vi "Process.vi"(8 "error in":errorcluster, 11 "MAUI":refnum<class "SMO.UI.MAUI.lvclass">) -> (0 "error out":errorcluster, 3 "MAUI out":refnum<class "SMO.UI.MAUI.lvclass">)   [LabVIEW 2020, in "SMO.UI.MAUI.lvclass"]
doc: "---------------------------------------------------------------\nJKI State Machine Objects™\nhttp://jki.net/state-machine-objects/\nCopyright (C) 2005-2015, JKI <info@jki.net>\nALL RIGHTS RESERVEDJKI State Machine Objects (SMO) 1.0.0.5\nJKI - JKI\nCopyright (c) 2016, JKI"
uses:
  SMO.UI.MAUI.lvclass
  C:/Program Files (x86)/National Instruments/LabVIEW 2020/vi.lib/JKI/JKI SMO/SMO/SMO.lvclass
  C:/Program Files (x86)/National Instruments/LabVIEW 2020/vi.lib/JKI/JKI SMO/SMO.UI/SMO.UI.lvclass
  <vilib>/JKI/JKI SMO/SMO/Typedefs/Parent Call--Enum.ctl
  Typedefs/DefaultSubpanel.ctl
  <vilib>/Levylab/SMO.UI.Embedded/SMO.UI.Embedded.lvclass
  SMO.UI.MAUI.lvclass/SMO.UI.MAUI.ctl
  <vilib>/Levylab/SMO.UI.Embedded/Typedefs/UI State.ctl
  Typedefs/PublicEvents--SMO.UI.MAUI.ReadyForInfo .ctl
  <vilib>/JKI/JKI SMO/SMO.UI/SMO.UI.lvclass
  <vilib>/JKI/JKI SMO/SMO/SMO.lvclass
panel:
  out "License":string="BSD 3-Clause License\n\nCopyright (c) 2020, Joseph Albro\nAll rights reserved.\n\nRedistribution and use in source and binary forms, with or without\nmodification, are permitted provided that the following conditions are met:\n\n1. Redistributions of source code must retain the above copyright notice, this\n   list of conditions and the following disclaimer.\n\n2. Redistributions in binary form must reproduce the above copyright notice,\n   this list of conditions and the following disclaimer in the documentation\n   and/or other materials provided with the distribution.\n\n3. Neither the name of the copyright holder nor the names of its\n   contributors may be used to endorse or promote products derived from\n   this software without specific prior written permission.\n\nTHIS SOFTWARE IS PROVIDED BY THE COPYRIGHT HOLDERS AND CONTRIBUTORS \"AS IS\"\nAND ANY EXPRESS OR IMPLIED WARRANTIES, INCLUDING, BUT NOT LIMITED TO, THE\nIMPLIED WARRANTIES OF MERCHANTABILITY AND FITNESS FOR A PARTICULAR PURPOSE ARE\nDISCLAIMED. IN NO EVENT SHALL THE COPYRIGHT HOLDER OR CONTRIBUTORS BE LIABLE\nFOR ANY DIRECT, INDIRECT, INCIDENTAL, SPECIAL, EXEMPLARY, OR CONSEQUENTIAL\nDAMAGES (INCLUDING, BUT NOT LIMITED TO, PROCUREMENT OF SUBSTITUTE GOODS OR\nSERVICES; LOSS OF USE, DATA, OR PROFITS; OR BUSINESS INTERRUPTION) HOWEVER\nCAUSED AND ON ANY THEORY OF LIABILITY, WHETHER IN CONTRACT, STRICT LIABILITY,\nOR TORT (INCLUDING NEGLIGENCE OR OTHERWISE) ARISING IN ANY WAY OUT OF THE USE\nOF THIS SOFTWARE, EVEN IF ADVISED OF THE POSSIBILITY OF SUCH DAMAGE."
  # "For instructions on how to use the JKI State Machine Objects, examples and video tutorials, visit:\nhttp://jki.net/state-machine-objects/\n\nJKI State Machine Objects™\nhttp://jki.net/state-machine-objects/\nCopyright (C) 2005-2015, JKI <info@jki.net>\nALL RIGHTS RESERVED"
  # "SMO.UI.MAUI"
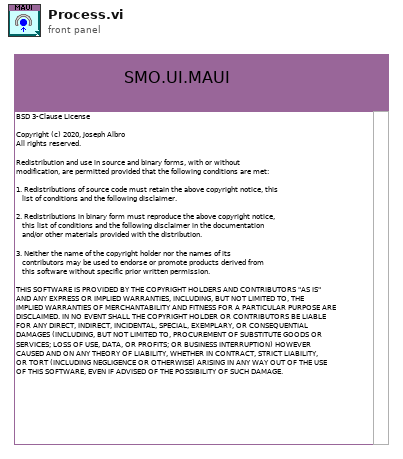
[diagram p1: front panel]
types:
  T1 = typedef "SMO.lvclass/Parent Call--Enum.ctl" = enum16{"Allows parent to run", "Does not request parent to run"}
  T2 = typedef "SMO.UI.MAUI.lvclass/DefaultSubpanel.ctl" = cluster{"SMO.UI.Embedded":refnum<class "SMO.UI.Embedded.lvclass">}
  T3 = enum32{"invalid app kind", "Development System", "Run Time System", "Student Edition", "Embedded LabVIEW", "Evaluation", "Custom"}
  T4 = enum32{"Invalid", "Standard", "Closed", "Hidden", "Minimized", "Maximized"}
  T5 = typedef "SMO.UI.MAUI.lvclass/PublicEvents--SMO.UI.MAUI.ReadyForInfo .ctl" = bool
  T6 = typedef "SMO.UI.MAUI.lvclass/PrivateEvents--SMO.UI.MAUI.GetDefaultSubpanel.ctl" = refnum<notifier>
  T7 = cluster{"SMO.UI.Embedded":refnum<class "SMO.UI.Embedded.lvclass">}
  T8 = typedef "SMO.UI.Embedded.lvclass/UI State.ctl" = enum16{"unknown", "Opened", "Embedded", "Closed"}
  T9 = cluster{"Core":cluster{"Current VI Reference":refnum<vi>, "Close Panel on Exit?":bool, "error":errorcluster}, "Self Reference":refnum<class "SMO.UI.MAUI.lvclass">, "Active Index":i32[], "Panel Index":i32[], "UI State":T8, "PopSubpanel":i32}
  T10 = typedef "SMO.UI.MAUI.lvclass/PrivateEvents--SMO.UI.MAUI.OpenSubpanel.ctl" = i32
  T11 = typedef "SMO.UI.MAUI.lvclass/PrivateEvents--SMO.UI.MAUI.SetPanelData.ctl" = T12[]
  T12 = typedef "SMO.UI.MAUI.lvclass/PanelData.ctl" = cluster{"SubPanel":refnum<vi>, "Ring":refnum<vi>, "Active":i32}
  T13 = typedef "SMO.UI.MAUI.lvclass/PrivateEvents--SMO.UI.MAUI.GetPanelData.ctl" = refnum<notifier>
  T14 = cluster{"Current VI Reference":refnum<vi>, "Close Panel on Exit?":bool, "error":errorcluster}
  T15 = typedef "SMO.lvclass/Protected Events.ctl" = cluster{"StopProcesses":refnum<user-event>, "AbortProcesses":refnum<user-event>, "Config Changed":refnum<user-event>, "Dependency":refnum<user-event>}
  T16 = typedef "SMO.UI.MAUI.lvclass/PrivateEvents--Cluster.ctl" = cluster{"SetEmbedded":refnum<user-event>, "GetEmbedded":refnum<user-event>, "SetPanelData":refnum<user-event>, "GetPanelData":refnum<user-event>, "UpdatePanel":refnum<user-event>, "PopSubpanel":refnum<user-event>, "GetDefaultSubpanel":refnum<user-event>, "SetDefaultSubpanel":refnum<user-event>}
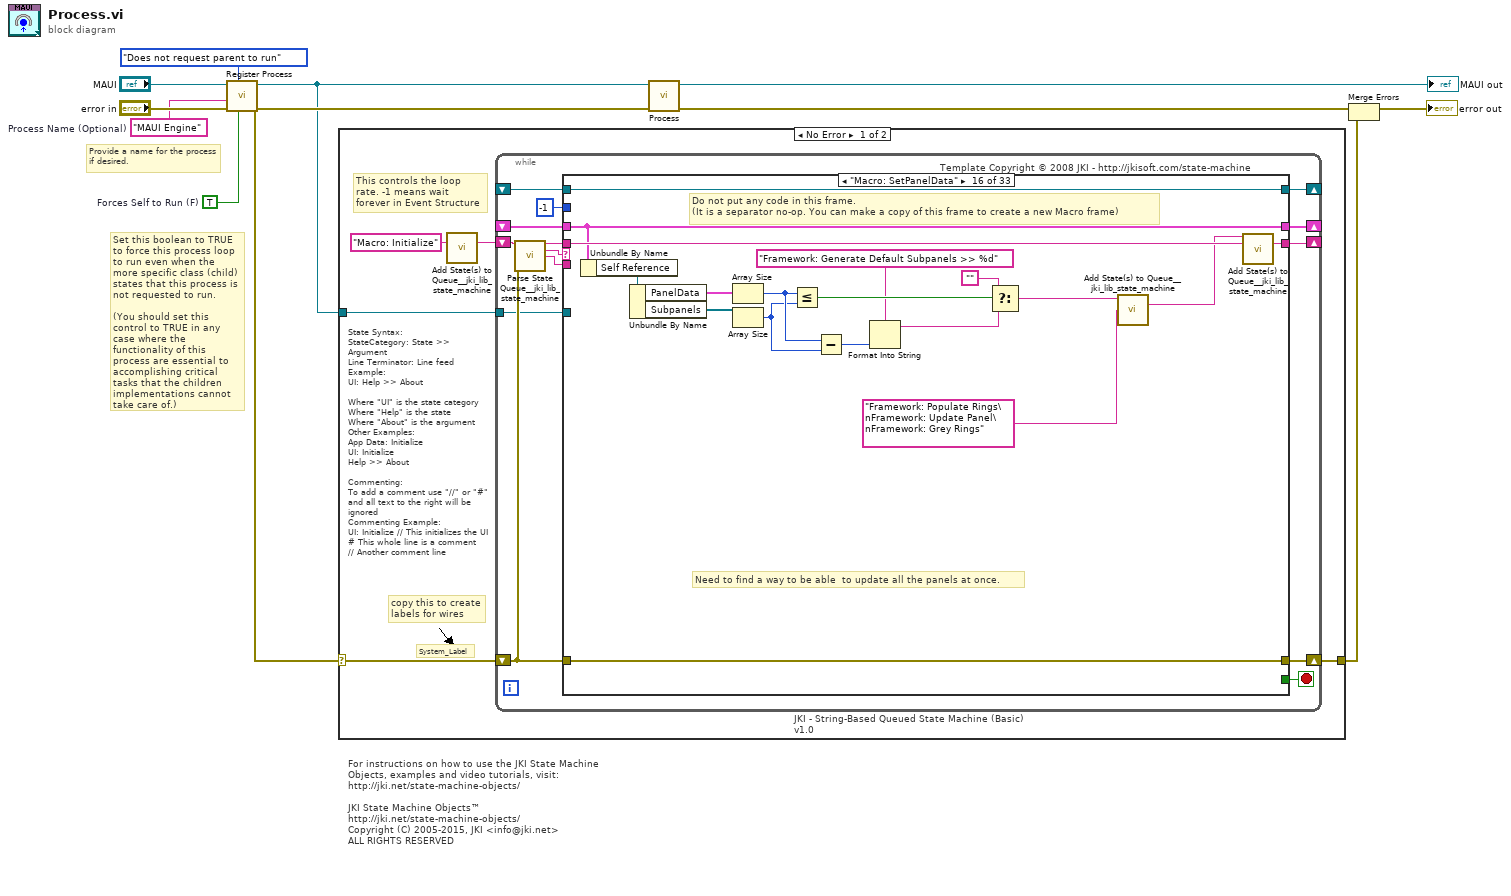
[diagram p0: block diagram]
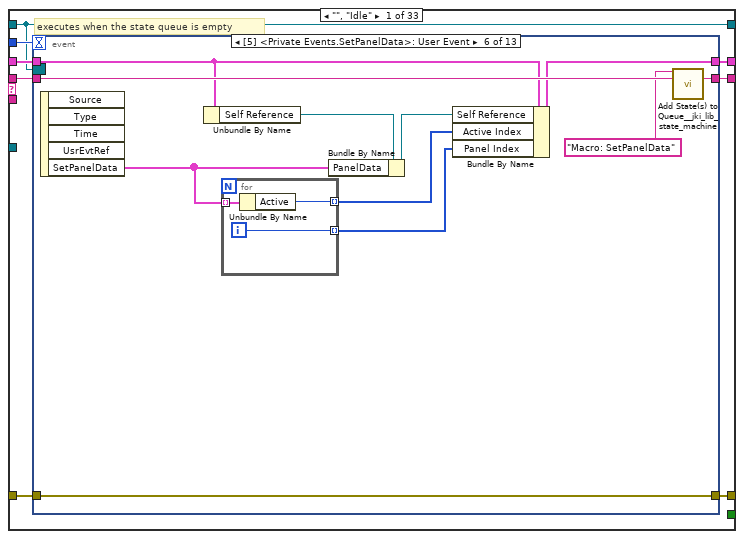
[diagram p2: hidden frame]
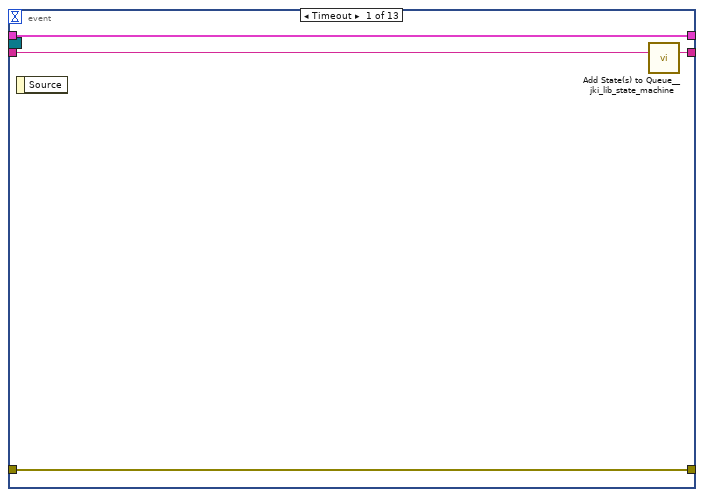
[diagram p3: hidden frame]
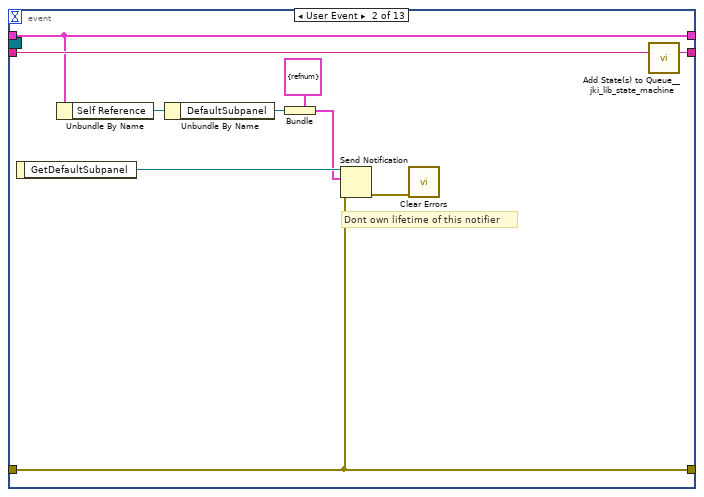
[diagram p4: hidden frame]
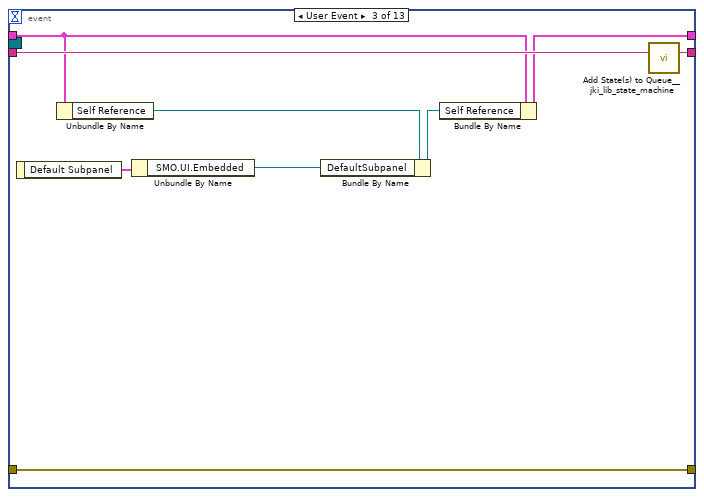
[diagram p5: hidden frame]
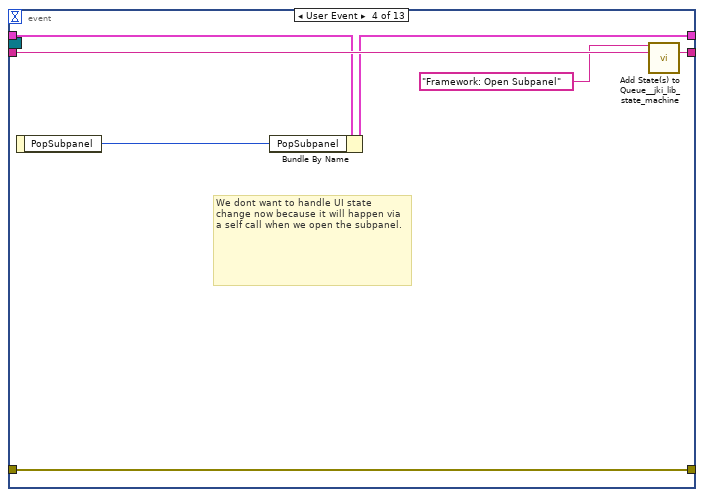
[diagram p6: hidden frame]
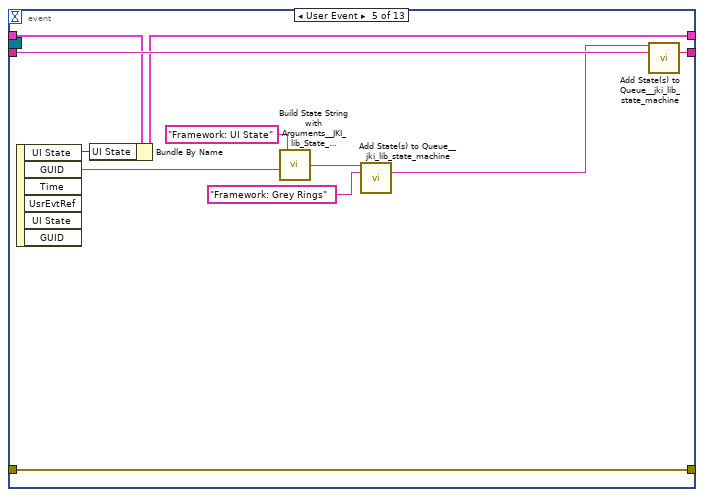
[diagram p7: hidden frame]
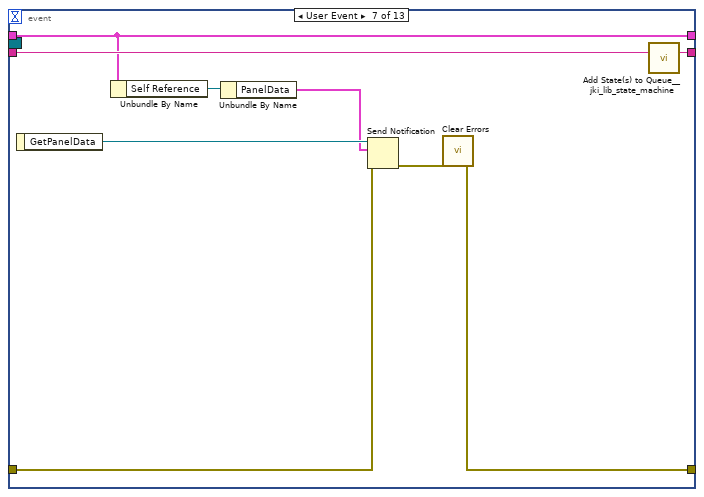
[diagram p8: hidden frame]
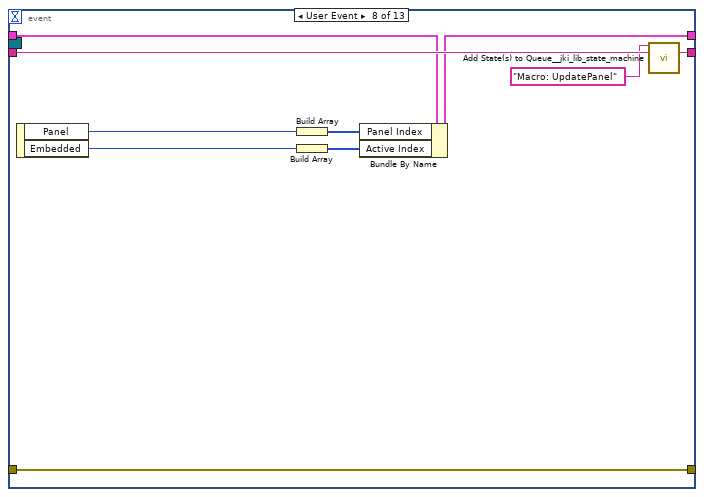
[diagram p9: hidden frame]
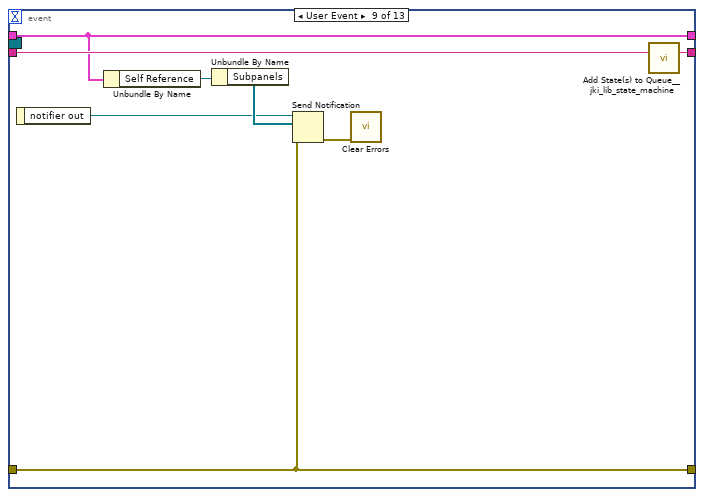
[diagram p10: hidden frame]
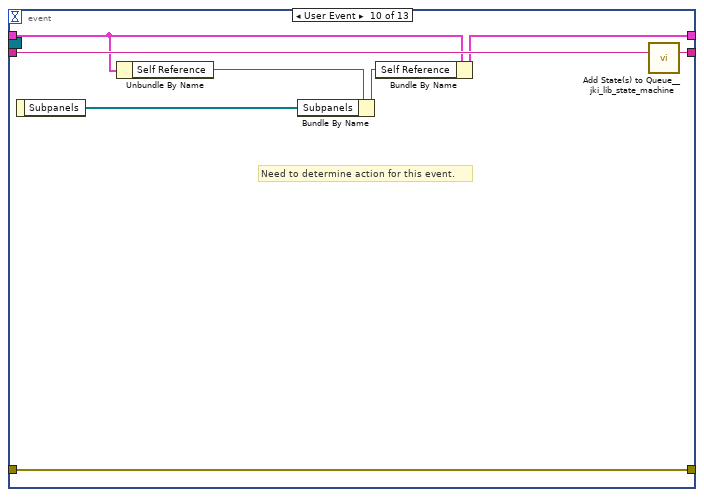
[diagram p11: hidden frame]
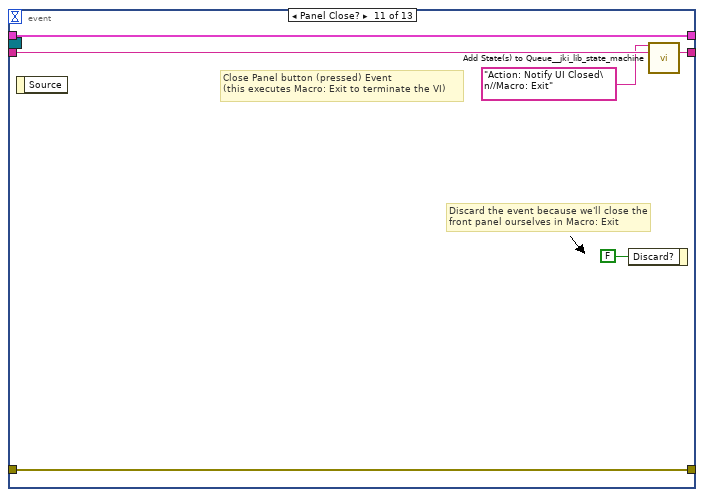
[diagram p12: hidden frame]
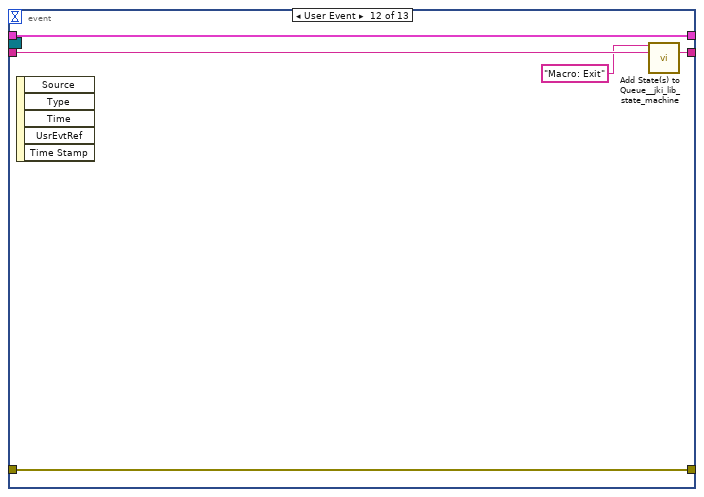
[diagram p13: hidden frame]
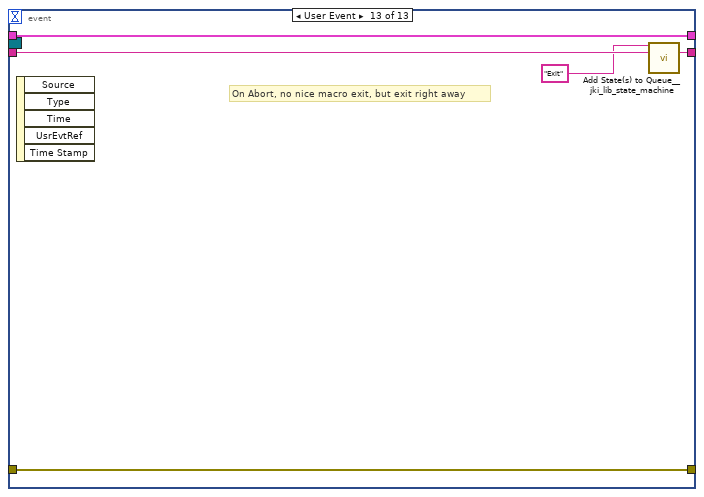
[diagram p14: hidden frame]
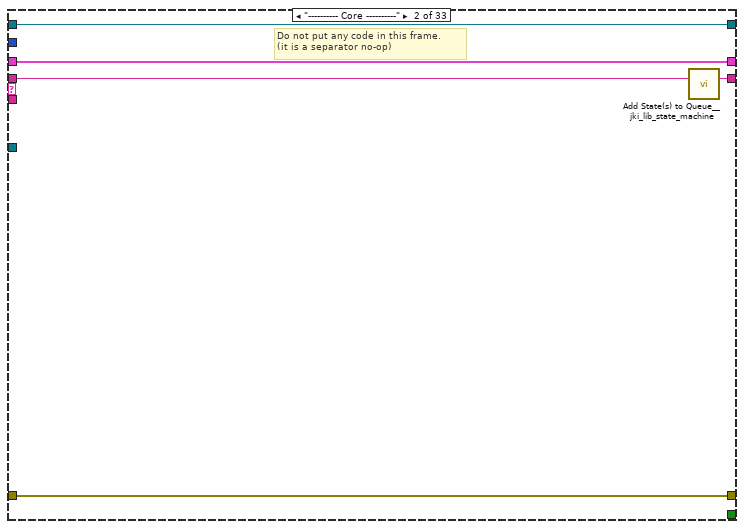
[diagram p15: hidden frame]
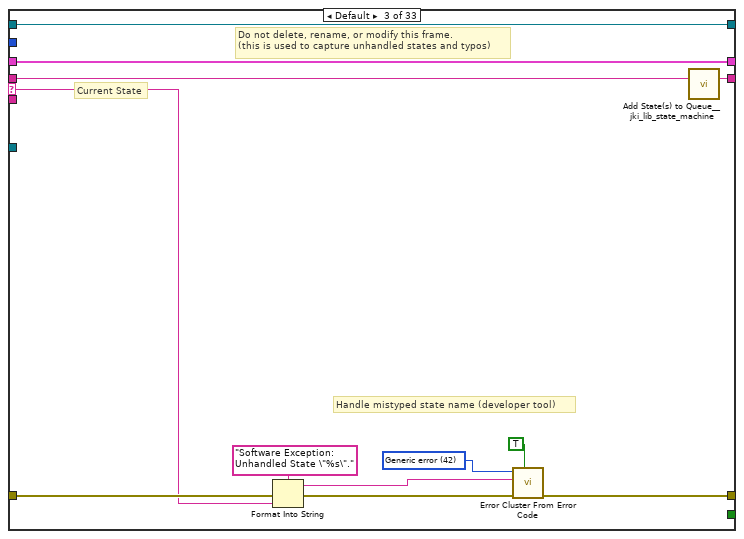
[diagram p16: hidden frame]
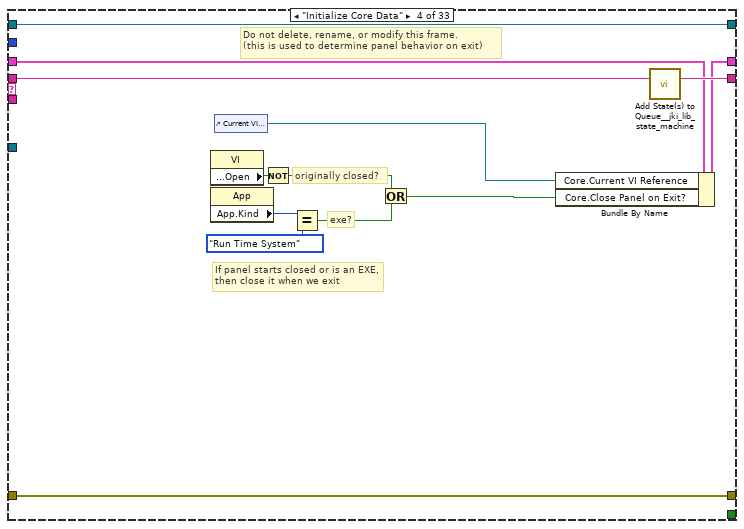
[diagram p17: hidden frame]
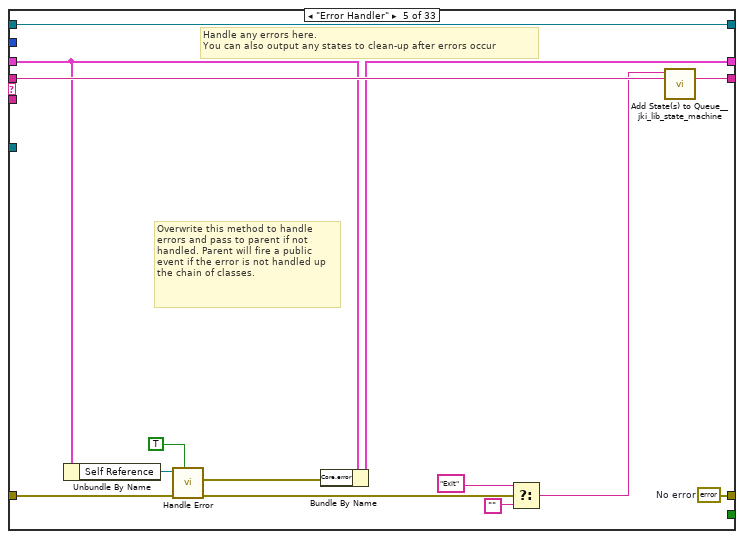
[diagram p18: hidden frame]
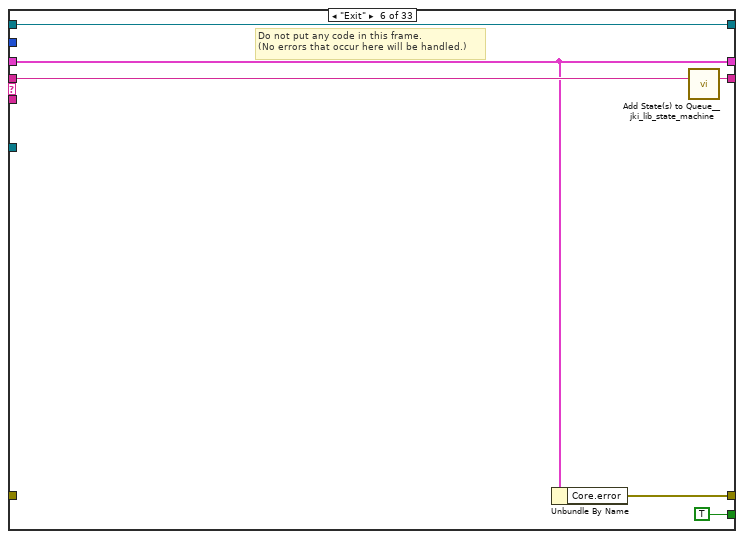
[diagram p19: hidden frame]
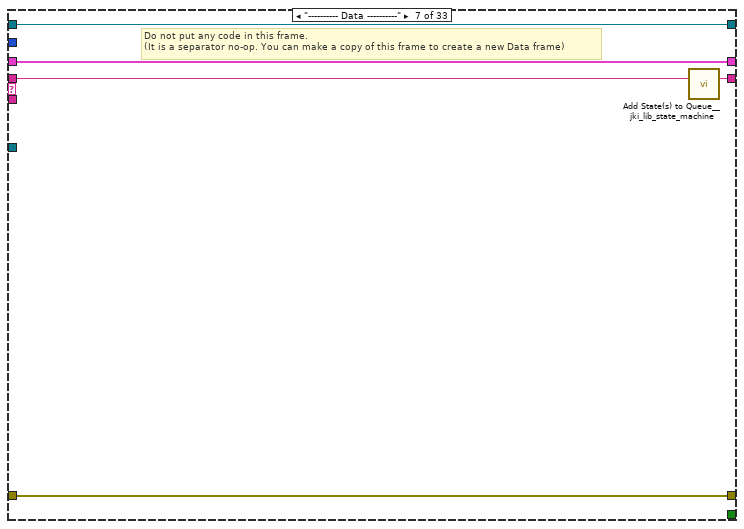
[diagram p20: hidden frame]
diagram:
  w2 = TRUE  # Forces Self to Run (F)
  w1 = "MAUI Engine"  # Process Name (Optional)
  # "Provide a name for the process\nif desired."
  # "Set this boolean to TRUE to force this process loop to run even when the more specific class (child) states that this process is not requested to run.\n\n(You should set this control to TRUE in any case where the functionality of this process are essential to accomplishing critical tasks that the children implementations cannot take care of.)"
  # "For instructions on how to use the JKI State Machine Objects, examples and video tutorials, visit:\nhttp://jki.net/state-machine-objects/\n\nJKI State Machine Objects™\nhttp://jki.net/state-machine-objects/\nCopyright (C) 2005-2015, JKI <info@jki.net>\nALL RIGHTS RESERVED"
  n1 = call <vilib>:"Register Process.vi"("Forces Self to Run (F)"=w2, "Parent Call"=Parent_Call--Enum."Does not request parent to run", "error in (no error)"="error in", "Process Name (optional)"=w1, "SMO"="MAUI") -> ("error out"=w8:errorcluster, "SMO out"=w7:refnum<class "SMO.UI.MAUI.lvclass">)  [unwired: 5 in]
  n2 = case shown="No Error" w8 {
    selector: w8 -> [w13 w484]
    tunnel: w7 -> [w14 _]
    tunnel: [w12 w484] -> w4
    frame No Error {
      # "State Syntax:\nStateCategory: State >> Argument\nLine Terminator: Line feed\nExample:\nUI: Help >> About\n\nWhere \"UI\" is the state category\nWhere \"Help\" is the state\nWhere \"About\" is the argument\nOther Examples:\nApp Data: Initialize\nUI: Initialize\nHelp >> About\n\nCommenting:\nTo add a comment use \"//\" or \"#\" and all text to the right will be ignored\nCommenting Example:\nUI: Initialize // This initializes the UI\n# This whole line is a comment\n// Another comment line"
      # "copy this to create labels for wires"
      # "This controls the loop rate. -1 means wait forever in Event Structure"
      # "System_Label"
      n3 = call <vilib>:"Add State(s) to Queue__jki_lib_state_machine.vi"("State(s) in (\"\")"="Macro: Initialize") -> ("States Out"=w16:string)  [unwired: 14 in]
      n4 = while "JKI - String-Based Queued State Machine (Basic) v1.0" {
        shift-right: [w23] -> _
        shift-left: _ -> [w22]
        shift-right: [w26] -> w12
        shift-left: w13 -> [w20]
        shift-right: [w25] -> _
        shift-left: w16 -> [w27]
        tunnel: w14 -> [w19]
        shift-right: [w18] -> _
        shift-left: _ -> [w17]
        stop <- w24 stop-if-true
        # "Template Copyright © 2008 JKI - http://jkisoft.com/state-machine"
        n5 = call <vilib>:"Parse State Queue__jki_lib_state_machine.vi"("State Queue"=w27, "Error In (no error)"=w20) -> ("Remaining States"=w29:string, "Current State"=w30:string, "Arguments"=w28:string)  [unwired: 11 in]
        n6 = case shown="\"Macro: SetPanelData\"" w30 {
          selector: w30 -> [_ _ w151 _ _ _ _ _ _ _ _ _ _ _ _ _ _ _ _ _ _ _ _ _ _ _ _ _ _ _ _ _ _]
          tunnel: w29 -> [w38 w149 w155 w174 w188 w194 w199 w213 w220 w225 w231 w238 w254 w286 w292 w310 w319 w333 w338 w349 w354 w367 w373 w380 w390 w397 w402 w419 w437 w448 w459 w474 w483]
          tunnel: w28 -> [_ _ _ _ _ _ _ _ _ _ _ w232 w248 _ _ _ _ _ _ _ _ _ _ _ _ _ _ w411 _ w444 _ _ _]
          tunnel: w22 -> [w36 w146 w153 w165 w177 w190 w196 _ w215 w222 w229 w236 w250 w283 w289 w306 w315 w324 w335 w346 w351 w365 w371 w376 w387 w393 w399 w414 w425 w439 w455 w467 w479]
          tunnel: [w35 w147 w157 w171 w179 w189 w197 w209 w216 w223 w228 w233 w251 w284 w290 w308 w317 w331 w336 w340 w352 w360 w368 w377 w382 w391 w400 w403 w428 w442 w451 w469 w475] -> w26
          tunnel: w20 -> [w34 w147 w156 w171 w184 _ w197 w210 w217 w223 w228 w234 w252 w284 w290 w308 w317 w331 w336 w341 w352 w362 w369 w377 w383 w392 w400 w413 w427 w441 w452 w470 w476]
          tunnel: [w37 w148 w154 w173 w187 w193 w198 w212 w219 w224 w230 w237 w253 w285 w291 w309 w318 w332 w337 w348 w353 w366 w372 w379 w389 w396 w401 w418 w436 w447 w458 w473 w482] -> w25
          tunnel: [_ _ _ _ _ TRUE _ _ _ _ _ _ _ _ _ _ _ _ _ _ _ _ _ _ _ _ _ _ _ _ _ _ _] -> w24
          tunnel: [w33 w146 w153 w172 w176 w190 w196 w211 w215 w222 w229 w236 w250 w283 w289 w306 w315 w324 w335 w346 w351 w365 w371 w375 w386 w393 w399 w415 w426 w440 w454 w466 w478] -> w23
          tunnel: -1 ("Timeout") -> [w32 _ _ _ _ _ _ _ _ _ _ _ _ _ _ _ _ _ _ _ _ _ _ _ _ _ _ _ _ _ _ _ _]
          tunnel: w19 -> [_ _ _ _ _ _ _ w207 _ _ _ _ _ _ _ _ _ _ _ _ _ _ _ _ _ _ _ _ _ _ _ _ _]
          tunnel: [w31 w145 w150 w162 w186 w191 w195 w205 w214 w221 w227 w235 w247 w282 w288 w307 w316 w325 w334 w347 w350 w364 w370 w378 w388 w395 w398 w417 w435 w446 w457 w472 w481] -> w18
          tunnel: w17 -> [w31 w145 w150 w162 w186 w191 w195 w205 w214 w221 w227 w235 w247 w282 w288 w307 w316 w325 w334 w347 w350 _ w370 w378 w388 w395 w398 w417 w435 w446 w457 w472 w481]
          frame "", "Idle" {
            # "executes when the state queue is empty"
            n7 = event shown="[5] <Private Events.SetPanelData>: User Event" {
              selector: w31 -> [_ _ _ _ _ _ _ _ _ _ _ _ _]
              dyn-events: _ -> [_ _ _ _ _ _ _ _ _ _ _ _ _]
              timeout: w32 -> [_ _ _ _ _ _ _ _ _ _ _ _ _]
              tunnel: w38 -> [w42 w52 w61 w68 w79 w90 w102 w112 w120 w128 w134 w139 w144]
              tunnel: [w41 w51 w60 w67 w78 w89 w101 w111 w119 w127 w133 w138 w143] -> w37
              tunnel: w36 -> [w39 w43 w57 w63 w75 w87 w99 w109 w118 w124 w130 w136 w141]
              tunnel: [w40 w46 w59 w66 w77 w88 w94 w110 w114 w126 w129 w137 w142] -> w35
              tunnel: w34 -> [w40 w46 w59 w66 w77 w88 w95 w110 w114 w126 w129 w137 w142]
              tunnel: [w39 w43 w58 w64 w76 w86 w99 w108 w118 w123 w130 w136 w141] -> w33
              event Timeout {
                n8 = event-data() -> ()  [unwired: 1 in, 1 out]
                n9 = call <vilib>:"Add State(s) to Queue__jki_lib_state_machine.vi"("State(s) in (\"\")"=w42) -> ("States Out"=w41:string)  [unwired: 14 in]
              }
              event User Event {
                # "Dont own lifetime of this notifier"
                n10 = event-data() -> ("GetDefaultSubpanel"=w49:T6)  [unwired: 1 in]
                n11 = Unbundle By Name(w43) -> ("Self Reference"=w50:refnum<class "SMO.UI.MAUI.lvclass">)
                n12 = Unbundle By Name(w50) -> ("DefaultSubpanel"=w44:refnum<class "SMO.UI.Embedded.lvclass">)
                n13 = Bundle(cluster=T2 {"SMO.UI.Embedded"=refnum} ("Default Subpanel"), "SMO.UI.Embedded"=w44) -> (w47:T2)
                n14 = Send Notification(notification=w47, notifier=w49, error in (no error)=w46) -> (error out=w45:errorcluster)  [unwired: 1 out]
                n15 = call <vilib>:"Clear Errors.vi"("error in (no error)"=w45) -> ()  [unwired: 5 in, 2 out]
                n16 = call <vilib>:"Add State(s) to Queue__jki_lib_state_machine.vi"("State(s) in (\"\")"=w52) -> ("States Out"=w51:string)  [unwired: 14 in]
              }
              event User Event {
                n17 = event-data() -> ("Default Subpanel"=w54:T7)  [unwired: 1 in]
                n18 = Unbundle By Name(w57) -> ("Self Reference"=w56:refnum<class "SMO.UI.MAUI.lvclass">)
                n19 = Unbundle By Name(w54) -> ("SMO.UI.Embedded"=w53:refnum<class "SMO.UI.Embedded.lvclass">)
                n20 = Bundle By Name(cluster=w56, "DefaultSubpanel"=w53) -> (w55:refnum<class "SMO.UI.MAUI.lvclass">)
                n21 = Bundle By Name(cluster=w57, "Self Reference"=w55) -> (w58:T9)
                n22 = call <vilib>:"Add State(s) to Queue__jki_lib_state_machine.vi"("State(s) in (\"\")"=w61) -> ("States Out"=w60:string)  [unwired: 14 in]
              }
              event User Event {
                # "We dont want to handle UI state change now because it will happen via a self call when we open the subpanel."
                n23 = event-data() -> ("PopSubpanel"=w62:T10)  [unwired: 1 in]
                n24 = Bundle By Name(cluster=w63, "PopSubpanel"=w62) -> (w64:T9)
                n25 = call <vilib>:"Add State(s) to Queue__jki_lib_state_machine.vi"("State(s) in Front (\"\")"="Framework: Open Subpanel", "State(s) in (\"\")"=w68) -> ("States Out"=w67:string)  [unwired: 13 in]
              }
              event User Event {
                n26 = event-data() -> ("UI State"=w74:T8, "GUID"=w72:string)  [unwired: 1 in, 4 out]
                n27 = Bundle By Name(cluster=w75, "UI State"=w74) -> (w76:T9)
                n28 = call <vilib>:"Build State String with Arguments__JKI_lib_State_Machine.vi"("Arguments (\"\")"=w72, "State"="Framework: UI State" ("State(s) in Front (\"\")")) -> ("State with Arguments"=w70:string)  [unwired: 4 in]
                n29 = call <vilib>:"Add State(s) to Queue__jki_lib_state_machine.vi"("State(s) in Front (\"\")"=w70, "State(s) in (\"\")"="Framework: Grey Rings" ("State(s) in (\"\")")) -> ("States Out"=w71:string)  [unwired: 13 in]
                n30 = call <vilib>:"Add State(s) to Queue__jki_lib_state_machine.vi"("State(s) in Front (\"\")"=w71, "State(s) in (\"\")"=w79) -> ("States Out"=w78:string)  [unwired: 13 in]
              }
              event User Event {
                n31 = event-data() -> ("SetPanelData"=w82:T11)  [unwired: 1 in, 4 out]
                n32 = Unbundle By Name(w87) -> ("Self Reference"=w85:refnum<class "SMO.UI.MAUI.lvclass">)
                n33 = for {
                  tunnel: w82 -> [w93] mode=indexing
                  tunnel: [w92] -> w81 mode=indexing
                  tunnel: [w91] -> w80 mode=indexing
                  i -> [w92]
                  n34 = Unbundle By Name(w93) -> ("Active"=w91:i32)
                }
                n35 = Bundle By Name(cluster=w85, "PanelData"=w82) -> (w84:refnum<class "SMO.UI.MAUI.lvclass">)
                n36 = Bundle By Name(cluster=w87, "Self Reference"=w84, "Active Index"=w80, "Panel Index"=w81) -> (w86:T9)
                n37 = call <vilib>:"Add State(s) to Queue__jki_lib_state_machine.vi"("State(s) in Front (\"\")"="Macro: SetPanelData", "State(s) in (\"\")"=w90) -> ("States Out"=w89:string)  [unwired: 13 in]
              }
              event User Event {
                n38 = event-data() -> ("GetPanelData"=w98:T13)  [unwired: 1 in]
                n39 = Unbundle By Name(w99) -> ("Self Reference"=w100:refnum<class "SMO.UI.MAUI.lvclass">)
                n40 = Unbundle By Name(w100) -> ("PanelData"=w97:T12[])
                n41 = Send Notification(notification=w97, notifier=w98, error in (no error)=w95) -> (error out=w96:errorcluster)  [unwired: 1 out]
                n42 = call <vilib>:"Clear Errors.vi"("error in (no error)"=w96) -> ("error out"=w94:errorcluster)  [unwired: 5 in, 1 out]
                n43 = call <vilib>:"Add State(s) to Queue__jki_lib_state_machine.vi"("State(s) in (\"\")"=w102) -> ("States Out"=w101:string)  [unwired: 14 in]
              }
              event User Event {
                n44 = event-data() -> ("Panel"=w106:i32, "Embedded"=w103:i32)  [unwired: 1 in]
                n45 = Build Array(w106) -> (w105:i32[])
                n46 = Build Array(w103) -> (w104:i32[])
                n47 = Bundle By Name(cluster=w109, "Panel Index"=w105, "Active Index"=w104) -> (w108:T9)
                n48 = call <vilib>:"Add State(s) to Queue__jki_lib_state_machine.vi"("State(s) in Front (\"\")"="Macro: UpdatePanel", "State(s) in (\"\")"=w112) -> ("States Out"=w111:string)  [unwired: 13 in]
              }
              event User Event {
                n49 = event-data() -> ("notifier out"=w115:refnum<notifier>)  [unwired: 1 in]
                n50 = Unbundle By Name(w118) -> ("Self Reference"=w117:refnum<class "SMO.UI.MAUI.lvclass">)
                n51 = Unbundle By Name(w117) -> ("Subpanels"=w116:refnum<class "SMO.UI.Embedded.lvclass">[])
                n52 = Send Notification(notification=w116, notifier=w115, error in (no error)=w114) -> (error out=w113:errorcluster)  [unwired: 1 out]
                n53 = call <vilib>:"Clear Errors.vi"("error in (no error)"=w113) -> ()  [unwired: 5 in, 2 out]
                n54 = call <vilib>:"Add State(s) to Queue__jki_lib_state_machine.vi"("State(s) in (\"\")"=w120) -> ("States Out"=w119:string)  [unwired: 14 in]
              }
              event User Event {
                # "Need to determine action for this event."
                n55 = event-data() -> ("Subpanels"=w121:refnum<class "SMO.UI.Embedded.lvclass">[])  [unwired: 1 in]
                n56 = Unbundle By Name(w124) -> ("Self Reference"=w125:refnum<class "SMO.UI.MAUI.lvclass">)
                n57 = Bundle By Name(cluster=w125, "Subpanels"=w121) -> (w122:refnum<class "SMO.UI.MAUI.lvclass">)
                n58 = Bundle By Name(cluster=w124, "Self Reference"=w122) -> (w123:T9)
                n59 = call <vilib>:"Add State(s) to Queue__jki_lib_state_machine.vi"("State(s) in (\"\")"=w128) -> ("States Out"=w127:string)  [unwired: 14 in]
              }
              event Panel Close? {
                # "Discard the event because we'll close the front panel ourselves in Macro: Exit"
                # "Close Panel button (pressed) Event\n(this executes Macro: Exit to terminate the VI)"
                n60 = event-data() -> ()  [unwired: 1 in, 1 out]
                n61 = event-data("Discard?"=FALSE) -> ()  [unwired: 1 in, 1 out]
                n62 = call <vilib>:"Add State(s) to Queue__jki_lib_state_machine.vi"("State(s) in Front (\"\")"="Action: Notify UI Closed\n//Macro: Exit", "State(s) in (\"\")"=w134) -> ("States Out"=w133:string)  [unwired: 13 in]
              }
              event User Event {
                n63 = event-data() -> ()  [unwired: 1 in, 5 out]
                n64 = call <vilib>:"Add State(s) to Queue__jki_lib_state_machine.vi"("State(s) in Front (\"\")"="Macro: Exit", "State(s) in (\"\")"=w139) -> ("States Out"=w138:string)  [unwired: 13 in]
              }
              event User Event {
                # "On Abort, no nice macro exit, but exit right away"
                n65 = event-data() -> ()  [unwired: 1 in, 5 out]
                n66 = call <vilib>:"Add State(s) to Queue__jki_lib_state_machine.vi"("State(s) in Front (\"\")"="Exit", "State(s) in (\"\")"=w144) -> ("States Out"=w143:string)  [unwired: 13 in]
              }
            }
          }
          frame "---------- Core ----------" {
            # "Do not put any code in this frame.\n(it is a separator no-op)"
            n67 = call <vilib>:"Add State(s) to Queue__jki_lib_state_machine.vi"("State(s) in (\"\")"=w149) -> ("States Out"=w148:string)  [unwired: 14 in]
          }
          frame Default {
            w160 = 42 items=["No error", "Argument error", "Memory is full", "Out of zone", "End of file", "File already open", "Generic file I/O error", "File not found", "File permission error", "Disk is full", "Duplicate path", "Too many files open", "System feature not enabled", "Resource file not found", "Cannot add resource", "Resource not found", "Image not found", "Image memory error", "Pen does not exist", "Config type invalid", "Config token not found", "Config parse error", "Config memory error", "Bad external code format", "Bad external code offset", "External code not present", "Null window", "Destroy window error", "Null menu", "Print aborted", "Bad print record", "Print driver error", "Windows error during printing", "Memory error during printing", "Print dialog error", "Generic print error", "Invalid device refnum", "Device not found", "Device parameter error", "Device unit error", "Cannot open device", "Device call aborted", "Generic error", "Cancelled by user", "Object ID too low", "Object ID too high", "Object not in heap", "Unknown heap", "Unknown object (invalid DefProc)", "Unknown object (DefProc not in table)", "Message out of range", "Invalid (null) method", "Unknown message", "Manager call not supported", "Bad address", "Network operation in progress", "Network operation timed out", "Connection is busy", "Network attribute not supported", "Network error", "Address in use", "System out of memory", "Connection aborted", "Connection refused", "Not connected", "Already connected", "Connection closed", "Initialization error (interapplication manager)", "Bad occurrence", "Wait on unbound occurrence handler", "Occurrence queue overflow", "Datalog type conflict", "Unused", "Unrecognized type (interapplication manager)", "Memory corrupt", "Failed to make temporary DLL", "Old CIN version", "Drag socket not found", "Failed to load drop-object", "Failed to register OLE object", "Failed to release OLE object", "Format specifier type mismatch", "Unknown format specifier", "Too few format specifiers", "Too many format specifiers", "Scan failed", "Newer CIN version", "Error converting to variant", "Runtime menu error", "Password tampered", "Variant attribute not found", "Incompatible variant data type", "Event data is not available", "Event Store is not present", "Occurrence is not found", "Event Queue is not created", "Event info is not available", "Refnum passed is NULL", "Error retrieving Class GUID", "Error retrieving CoClass GUID", "Error retrieving TypeLib GUID.", "Bad built application magic bytes.", "Specific driver is different from the specific driver associated with the Logical Name.", "There is no session opened to the class driver.", "Max Error", "MAX - Error with config objects", "MAX - Error loading configuration", "MAX - Group not supported"]
            # "Current State"
            # "Do not delete, rename, or modify this frame.\n(this is used to capture unhandled states and typos)"
            # "Handle mistyped state name (developer tool)"
            n68 = Format Into String(format string="Software Exception: Unhandled State \"%s\"." ("message"), error in=w156, w151) -> (resulting string=w159:string, error out=w158:errorcluster)  [unwired: 1 in]
            n69 = call <vilib>:"Error Cluster From Error Code.vi"("show call chain? (False)"=TRUE, "error in (no error)"=w158, "error message (\"\")"=w159, "error code (0)"=w160) -> ("error out"=w157:errorcluster)  [unwired: 5 in]
            n70 = call <vilib>:"Add State(s) to Queue__jki_lib_state_machine.vi"("State(s) in (\"\")"=w155) -> ("States Out"=w154:string)  [unwired: 14 in]
          }
          frame "Initialize Core Data" {
            # "Do not delete, rename, or modify this frame.\n(this is used to determine panel behavior on exit)"
            # "originally closed?"
            # "exe?"
            # "If panel starts closed or is an EXE, then close it when we exit"
            n71 = property class="VI"() -> ("Front Panel.Open"=w170:bool)  [unwired: 2 in, 2 out]
            n72 = property class="App"() -> ("App.Kind"=w169:T3)  [unwired: 2 in, 2 out]
            n73 = control-ref of="Current VI Reference"() -> (w163:refnum<vi>)
            n74 = Not(x=w170) -> (.not. x?=w167:bool)
            n75 = Equal?(x=w169, y=T3."Run Time System" ("Application:Kind")) -> (x = y?=w166:bool)
            n76 = Or(x=w167, y=w166) -> (x .or. y?=w164:bool)
            n77 = Bundle By Name(cluster=w165, "Core.Current VI Reference"=w163, "Core.Close Panel on Exit?"=w164) -> (w172:T9)
            n78 = call <vilib>:"Add State(s) to Queue__jki_lib_state_machine.vi"("State(s) in (\"\")"=w174) -> ("States Out"=w173:string)  [unwired: 14 in]
          }
          frame "Error Handler" {
            w179 = errorcluster {"status"=FALSE, "code"=0, "source"=""}  # No error
            # "Overwrite this method to handle errors and pass to parent if not handled. Parent will fire a public event if the error is not handled up the chain of classes."
            # "Handle any errors here.\nYou can also output any states to clean-up after errors occur"
            n79 = Unbundle By Name(w177) -> ("Self Reference"=w185:refnum<class "SMO.UI.MAUI.lvclass">)
            n80 = call-dynamic "Handle Error.vi"("Stop on Unhandled Error (T)"=TRUE, "error in"=w184, "SMO"=w185) -> ("handling error"=w180:errorcluster, "Unhandled error"=w178:errorcluster)  [unwired: 6 in, 1 out]
            n81 = Bundle By Name(cluster=w177, "Core.error"=w178) -> (w176:T9)
            n82 = Select(t="Exit", s=w180, f="") -> (s? t:f=w181:string)
            n83 = call <vilib>:"Add State(s) to Queue__jki_lib_state_machine.vi"("State(s) in Front (\"\")"=w181, "State(s) in (\"\")"=w188) -> ("States Out"=w187:string)  [unwired: 13 in]
          }
          frame "Exit" {
            # "Do not put any code in this frame.\n(No errors that occur here will be handled.)"
            n84 = Unbundle By Name(w190) -> ("Core.error"=w189:errorcluster)
            n85 = call <vilib>:"Add State(s) to Queue__jki_lib_state_machine.vi"("State(s) in (\"\")"=w194) -> ("States Out"=w193:string)  [unwired: 14 in]
          }
          frame "---------- Data ----------" {
            # "Do not put any code in this frame.\n(It is a separator no-op. You can make a copy of this frame to create a new Data frame)"
            n86 = call <vilib>:"Add State(s) to Queue__jki_lib_state_machine.vi"("State(s) in (\"\")"=w199) -> ("States Out"=w198:string)  [unwired: 14 in]
          }
          frame "Data: Initialize" {
            w200 = 0  # PopSubpanel
            w201 = UI_State."unknown"  # UI State
            w202 = i32[] []  # Panel Index
            w203 = i32[] []  # Active Index
            w204 = T14 {"Current VI Reference"=refnum, "Close Panel on Exit?"=FALSE, "error"={"status"=FALSE, "code"=0, "source"=""}}  # Core
            w208 = refnum<class "SMO.UI.MAUI.lvclass"> refnum  # Self Reference
            # "do not delete - used by framework"
            # "Expand Bundle to add new data elements to shift register data."
            # "Data names and types of shift register data are defined by this bundle."
            # "Initialize the shift-register data, here.\n(data names are defined by what you wire into the bundle function)"
            n87 = Variant To Data(error in=w210, type=w208, Variant=w207) -> (data=w206:refnum<class "SMO.UI.MAUI.lvclass">, error out=w209:errorcluster)
            n88 = Bundle("Core"=w204, "Self Reference"=w206, "Active Index"=w203, "Panel Index"=w202, "UI State"=w201, "PopSubpanel"=w200) -> (w211:T9)  [unwired: 1 in]
            n89 = call <vilib>:"Add State(s) to Queue__jki_lib_state_machine.vi"("State(s) in (\"\")"=w213) -> ("States Out"=w212:string)  [unwired: 14 in]
          }
          frame "Data: Cleanup" {
            # "Cleanup any data and references, here.\n(this is called automatically, by the Macro: Exit)"
            n90 = Unbundle By Name(w215) -> ("Core.Current VI Reference"=w218:refnum<vi>)
            n91 = Close Reference(reference=w218, error in (no error)=w217) -> (error out=w216:errorcluster)
            n92 = call <vilib>:"Add State(s) to Queue__jki_lib_state_machine.vi"("State(s) in (\"\")"=w220) -> ("States Out"=w219:string)  [unwired: 14 in]
          }
          frame "---------- UI ----------" {
            # "Do not put any code in this frame.\n(It is a separator no-op. You can make a copy of this frame to create a new UI frame)"
            n93 = call <vilib>:"Add State(s) to Queue__jki_lib_state_machine.vi"("State(s) in (\"\")"=w225) -> ("States Out"=w224:string)  [unwired: 14 in]
          }
          frame "UI: Initialize" {
            # "Initialize the User Interface, here.\n(this is called automatically, by the Macro: Init)"
            n94 = call <vilib>:"Add State(s) to Queue__jki_lib_state_machine.vi"("State(s) in (\"\")"=w231) -> ("States Out"=w230:string)  [unwired: 14 in]
            "License" <- "BSD 3-Clause License\n\nCopyright (c) 2020, Joseph Albro\nAll rights reserved.\n\nRedistribution and use in source and binary forms, with or without\nmodification, are permitted provided that the following conditions are met:\n\n1. Redistributions of source code must retain the above copyright notice, this\n   list of conditions and the following disclaimer.\n\n2. Redistributions in binary form must reproduce the above copyright notice,\n   this list of conditions and the following disclaimer in the documentation\n   and/or other materials provided with the distribution.\n\n3. Neither the name of the copyright holder nor the names of its\n   contributors may be used to endorse or promote products derived from\n   this software without specific prior written permission.\n\nTHIS SOFTWARE IS PROVIDED BY THE COPYRIGHT HOLDERS AND CONTRIBUTORS \"AS IS\"\nAND ANY EXPRESS OR IMPLIED WARRANTIES, INCLUDING, BUT NOT LIMITED TO, THE\nIMPLIED WARRANTIES OF MERCHANTABILITY AND FITNESS FOR A PARTICULAR PURPOSE ARE\nDISCLAIMED. IN NO EVENT SHALL THE COPYRIGHT HOLDER OR CONTRIBUTORS BE LIABLE\nFOR ANY DIRECT, INDIRECT, INCIDENTAL, SPECIAL, EXEMPLARY, OR CONSEQUENTIAL\nDAMAGES (INCLUDING, BUT NOT LIMITED TO, PROCUREMENT OF SUBSTITUTE GOODS OR\nSERVICES; LOSS OF USE, DATA, OR PROFITS; OR BUSINESS INTERRUPTION) HOWEVER\nCAUSED AND ON ANY THEORY OF LIABILITY, WHETHER IN CONTRACT, STRICT LIABILITY,\nOR TORT (INCLUDING NEGLIGENCE OR OTHERWISE) ARISING IN ANY WAY OUT OF THE USE\nOF THIS SOFTWARE, EVEN IF ADVISED OF THE POSSIBILITY OF SUCH DAMAGE."
          }
          frame "UI: Cursor Set" {
            # "Argument"
            # "Initialize the User Interface, here.\n(this is called automatically, by the Macro: Init)"
            n95 = disable-structure shown="Default" {
              disable-tunnel: w234 -> [w239 w242]
              disable-tunnel: [w239 w241] -> w233
              disable-tunnel: w232 -> [_ w240]
              frame condition #0 {
              }
              frame condition #1 (active) {
                n96 = case shown="\"Idle\", Default" w240 {
                  tunnel: w242 -> [w244 w246]
                  tunnel: [w243 w245] -> w241
                  frame "Idle", Default {
                    n97 = call <vilib>:"Unset Busy.vi"("error in (no error)"=w244) -> ("error out"=w243:errorcluster)  [unwired: 10 in]
                  }
                  frame "Busy" {
                    n98 = call <vilib>:"Set Busy.vi"("error in (no error)"=w246) -> ("error out"=w245:errorcluster)  [unwired: 9 in, 1 out]
                  }
                }
              }
            }
            n99 = call <vilib>:"Add State(s) to Queue__jki_lib_state_machine.vi"("State(s) in (\"\")"=w238) -> ("States Out"=w237:string)  [unwired: 14 in]
          }
          frame "UI: Front Panel State" {
            # "Argument"
            # "Set Front Panel Open or Closed\n(Usage: \"UI: Front Panel State >> Open|Close\")"
            n100 = Unbundle By Name(w250) -> ("Core.Current VI Reference"=w249:refnum<vi>)
            n101 = disable-structure shown="Default" {
              disable-tunnel: w252 -> [w258 w281]
              disable-tunnel: [w257 w281] -> w251
              disable-tunnel: w249 -> [w256 _]
              disable-tunnel: w248 -> [w255 _]
              frame condition #0 (active) {
                n102 = case shown="\"Close\"" w255 {
                  tunnel: w258 -> [w262 w275]
                  tunnel: [w264 w276] -> w257
                  tunnel: w256 -> [w263 w273]
                  frame "Open", Default {
                    n103 = property class="VI"(reference=w263, error in=w262) -> (reference out=w260:refnum<vi>, error out=w261:errorcluster, "FP.State"=w259:T4)
                    n104 = case shown="\"Closed\"" w259 {
                      tunnel: [w267 w270] -> w264
                      tunnel: w261 -> [w266 w270]
                      tunnel: w260 -> [w265 _]
                      frame "Closed" {
                        n105 = invoke class="VI" method="FP.Open"(reference=w265, error in=w266, "Activate"=TRUE, "State"=T4."Standard") -> (error out=w267:errorcluster)  [unwired: 1 in, 4 out]
                      }
                      frame Default {
                      }
                    }
                  }
                  frame "Close" {
                    n106 = property class="VI"(reference=w273, error in=w275) -> (reference out=w272:refnum<vi>, error out=w274:errorcluster, "FP.State"=w271:T4)
                    n107 = case shown="Default" w271 {
                      tunnel: [w277 w280] -> w276
                      tunnel: w274 -> [w277 w279]
                      tunnel: w272 -> [_ w278]
                      frame "Invalid", "Closed" {
                      }
                      frame Default {
                        n108 = invoke class="VI" method="FP.Close"(reference=w278, error in=w279) -> (error out=w280:errorcluster)  [unwired: 1 in, 2 out]
                      }
                    }
                  }
                }
              }
              frame condition #1 {
              }
            }
            n109 = call <vilib>:"Add State(s) to Queue__jki_lib_state_machine.vi"("State(s) in (\"\")"=w254) -> ("States Out"=w253:string)  [unwired: 14 in]
          }
          frame "---------- Macro ----------" {
            # "Do not put any code in this frame.\n(It is a separator no-op. You can make a copy of this frame to create a new Macro frame)"
            n110 = call <vilib>:"Add State(s) to Queue__jki_lib_state_machine.vi"("State(s) in (\"\")"=w286) -> ("States Out"=w285:string)  [unwired: 14 in]
          }
          frame "Macro: UpdatePanel" {
            # "Do not put any code in this frame.\n(It is a separator no-op. You can make a copy of this frame to create a new Macro frame)"
            n111 = call <vilib>:"Add State(s) to Queue__jki_lib_state_machine.vi"("State(s) in Front (\"\")"="Framework: Update Panel\nFramework: Grey Rings", "State(s) in (\"\")"=w292) -> ("States Out"=w291:string)  [unwired: 13 in]
          }
          frame "Macro: SetPanelData" {
            # "Need to find a way to be able  to update all the panels at once."
            # "Do not put any code in this frame.\n(It is a separator no-op. You can make a copy of this frame to create a new Macro frame)"
            n112 = Unbundle By Name(w306) -> ("Self Reference"=w305:refnum<class "SMO.UI.MAUI.lvclass">)
            n113 = Unbundle By Name(w305) -> ("PanelData"=w303:T12[], "Subpanels"=w304:refnum<class "SMO.UI.Embedded.lvclass">[])
            n114 = Array Size(array=w303) -> (size(s)=w301:i32)
            n115 = Array Size(array=w304) -> (size(s)=w300:i32)
            n116 = Less Or Equal?(x=w301, y=w300) -> (x <= y?=w302:bool)
            n117 = Subtract(x=w301, y=w300) -> (x-y=w299:i32)
            n118 = Format Into String(format string="Framework: Generate Default Subpanels >> %d", w299) -> (resulting string=w294:string)  [unwired: 2 in, 1 out]
            n119 = Select(t="", s=w302, f=w294) -> (s? t:f=w297:string)
            n120 = call <vilib>:"Add State(s) to Queue__jki_lib_state_machine.vi"("State(s) in Front (\"\")"=w297, "State(s) at Back (\"\")"="Framework: Populate Rings\nFramework: Update Panel\nFramework: Grey Rings") -> ("States Out"=w295:string)  [unwired: 13 in]
            n121 = call <vilib>:"Add State(s) to Queue__jki_lib_state_machine.vi"("State(s) in Front (\"\")"=w295, "State(s) in (\"\")"=w310) -> ("States Out"=w309:string)  [unwired: 13 in]
          }
          frame "Macro: Initialize" {
            w313 = "UI: Initialize\n//UI: Front Panel State >> Open\nAction: Notify Ready for Info"  # UI: Initialize //UI: Front Panel State >> Open Action: Notify Ready for Info
            # "Initialization Macro\n(This is called once, when the VI starts)"
            n122 = call <vilib>:"Add State(s) to Queue__jki_lib_state_machine.vi"("State(s) in Front (\"\")"="Data: Initialize\nInitialize Core Data\nEvents: Register", "State(s) in (\"\")"="Process: Sync", "State(s) at Back (\"\")"=w313) -> ("States Out"=w312:string)  [unwired: 12 in]
            n123 = call <vilib>:"Add State(s) to Queue__jki_lib_state_machine.vi"("State(s) in Front (\"\")"=w312, "State(s) in (\"\")"=w319) -> ("States Out"=w318:string)  [unwired: 13 in]
          }
          frame "Macro: Exit" {
            # "Exit Macro\n(This is called once, when the VI exits)"
            n124 = Unbundle By Name(w324) -> ("Core.Close Panel on Exit?"=w330:bool)
            n125 = Select(t="//UI: Front Panel State >> Close", s=w330, f="") -> (s? t:f=w327:string)
            n126 = call <vilib>:"Add State(s) to Queue__jki_lib_state_machine.vi"("State(s) in Front (\"\")"="Data: Cleanup\nEvents: Unregister", "State(s) in (\"\")"="Process: Sync", "State(s) at Back (\"\")"="Exit") -> ("States Out"=w321:string)  [unwired: 12 in]
            n127 = call <vilib>:"Add State(s) to Queue__jki_lib_state_machine.vi"("State(s) in (\"\")"=w327, "State(s) at Back (\"\")"=w321) -> ("States Out"=w326:string)  [unwired: 13 in]
            n128 = call <vilib>:"Add State(s) to Queue__jki_lib_state_machine.vi"("State(s) in Front (\"\")"=w326, "State(s) in (\"\")"=w333) -> ("States Out"=w332:string)  [unwired: 13 in]
          }
          frame "---------- Process ----------" {
            # "Template Separator\n(You can make a copy of, or modify, this frame)"
            n129 = call <vilib>:"Add State(s) to Queue__jki_lib_state_machine.vi"("State(s) in (\"\")"=w338) -> ("States Out"=w337:string)  [unwired: 14 in]
          }
          frame "Process: Sync" {
            n130 = Unbundle By Name(w346) -> ("Self Reference"=w342:refnum<class "SMO.UI.MAUI.lvclass">)
            n131 = call <vilib>:"WaitOnProcessSync.vi"("error in (no error)"=w341, "SMO"=w342) -> ("error out"=w340:errorcluster, "Don't run?"=w345:bool)  [unwired: 7 in, 1 out]
            n132 = Select(t="Data: Cleanup\nEvents: Unregister\nExit", s=w345, f="") -> (s? t:f=w339:string)
            n133 = call <vilib>:"Add State(s) to Queue__jki_lib_state_machine.vi"("State(s) in Front (\"\")"=w339, "State(s) in (\"\")"=w349) -> ("States Out"=w348:string)  [unwired: 13 in]
          }
          frame "---------- Events ----------" {
            # "Template Separator\n(You can make a copy of, or modify, this frame)"
            n134 = call <vilib>:"Add State(s) to Queue__jki_lib_state_machine.vi"("State(s) in (\"\")"=w354) -> ("States Out"=w353:string)  [unwired: 14 in]
          }
          frame "Events: Register" {
            # "Expand to add\nmore events"
            # "Base Class Protected Events"
            n135 = Unbundle By Name(w365) -> ("Self Reference"=w356:refnum<class "SMO.UI.MAUI.lvclass">)
            n136 = call <vilib>:"GetProtectedEvents.vi"("SMO"=w356) -> ("error out"=w359:errorcluster, "SMO Protected Events"=w363:T15)  [unwired: 8 in, 1 out]
            n137 = call "GetAllUIStateChange.vi"("SMO.UI.MAUI in"=w356) -> ("UIState"=w355:refnum<user-event>[])  [unwired: 8 in, 2 out]
            n138 = call "SMO.UI.MAUI.GetPrivateEvents.vi"("MAUI"=w356) -> ("error out"=w357:errorcluster, "Private Events"=w358:T16)  [unwired: 8 in, 1 out]
            n139 = register-events(w363, w358, w355) -> (reference out=w364:refnum<event-registration>, error out=w361:errorcluster)  [unwired: 2 in]
            n140 = Merge Errors(w362, w361, w359, w357) -> (w360:errorcluster)
            n141 = call <vilib>:"Add State(s) to Queue__jki_lib_state_machine.vi"("State(s) in (\"\")"=w367) -> ("States Out"=w366:string)  [unwired: 14 in]
          }
          frame "Events: Unregister" {
            n142 = Unregister For Events(event registration refnum=w370, error in=w369) -> (error out=w368:errorcluster)
            n143 = call <vilib>:"Add State(s) to Queue__jki_lib_state_machine.vi"("State(s) in (\"\")"=w373) -> ("States Out"=w372:string)  [unwired: 14 in]
          }
          frame "---------- Action ----------" {
            n144 = Unbundle By Name(w376) -> ("Self Reference"=w374:refnum<class "SMO.UI.MAUI.lvclass">)
            n145 = Bundle By Name(cluster=w376, "Self Reference"=w374) -> (w375:T9)
            n146 = call <vilib>:"Add State(s) to Queue__jki_lib_state_machine.vi"("State(s) in (\"\")"=w380) -> ("States Out"=w379:string)  [unwired: 14 in]
          }
          frame "Action: Notify Ready for Info" {
            n147 = Unbundle By Name(w387) -> ("Self Reference"=w385:refnum<class "SMO.UI.MAUI.lvclass">)
            n148 = call "SMO.UI.MAUI.ReadyForInfo.vi"("error in (no error)"=w383, "ReadyForInfo"=T5 TRUE, "MAUI"=w385) -> ("error out"=w382:errorcluster, "MAUI out"=w384:refnum<class "SMO.UI.MAUI.lvclass">)  [unwired: 7 in]
            n149 = Bundle By Name(cluster=w387, "Self Reference"=w384) -> (w386:T9)
            n150 = call <vilib>:"Add State(s) to Queue__jki_lib_state_machine.vi"("State(s) in (\"\")"=w390) -> ("States Out"=w389:string)  [unwired: 14 in]
          }
          frame "Action: Notify UI Closed" {
            # "Notify that the UI has been closed"
            n151 = Unbundle By Name(w393) -> ("Self Reference"=w394:refnum<class "SMO.UI.MAUI.lvclass">)
            n152 = call <vilib>:"Hide.vi"("error in (no error)"=w392, "SMO.UI"=w394) -> ("error out"=w391:errorcluster)  [unwired: 8 in, 1 out]
            n153 = call <vilib>:"Add State(s) to Queue__jki_lib_state_machine.vi"("State(s) in (\"\")"=w397) -> ("States Out"=w396:string)  [unwired: 14 in]
          }
          frame "---------- Framework ----------" {
            # "Template Separator\n(You can make a copy of, or modify, this frame)"
            n154 = call <vilib>:"Add State(s) to Queue__jki_lib_state_machine.vi"("State(s) in (\"\")"=w402) -> ("States Out"=w401:string)  [unwired: 14 in]
          }
          frame "Framework: Generate Default Subpanels" {
            # "Wouldnt let me put this in the inner method?"
            # "Template Separator\n(You can make a copy of, or modify, this frame)"
            n155 = Unbundle By Name(w414) -> ("Self Reference"=w416:refnum<class "SMO.UI.MAUI.lvclass">)
            n156 = Decimal String To Number(string=w411) -> (number=w412:i32)  [unwired: 2 in, 1 out]
            n157 = call "GenerateDefaultSubpanels.vi"("error in (no error)"=w413, "Number"=w412, "SMO.UI.MAUI in"=w416) -> ("error out"=w404:errorcluster, "Array"=w410:refnum<class "SMO.UI.Embedded.lvclass">[], "SMO.UI.MAUI out"=w407:refnum<class "SMO.UI.MAUI.lvclass">)  [unwired: 6 in]
            n158 = Unbundle By Name(w407) -> ("Subpanels"=w409:refnum<class "SMO.UI.Embedded.lvclass">[])
            n159 = for {
              tunnel: w410 -> [w423] mode=indexing
              shift-right: [w421] -> w403
              shift-left: w404 -> [w422]
              tunnel: [w420] -> w408 mode=indexing
              n160 = call <vilib>:"Start.vi"("error in (no error)"=w422, "SMO"=w423) -> ("error out"=w421:errorcluster, "SMO out"=w420:refnum<class "SMO.UI.Embedded.lvclass">)  [unwired: 8 in]
            }
            n161 = Build Array (concatenate)(w409, w408) -> (w405:refnum<class "SMO.UI.Embedded.lvclass">[])
            n162 = Bundle By Name(cluster=w407, "Subpanels"=w405) -> (w406:refnum<class "SMO.UI.MAUI.lvclass">)
            n163 = Bundle By Name(cluster=w414, "Self Reference"=w406) -> (w415:T9)
            n164 = call <vilib>:"Add State(s) to Queue__jki_lib_state_machine.vi"("State(s) in (\"\")"=w419) -> ("States Out"=w418:string)  [unwired: 14 in]
          }
          frame "Framework: Open Subpanel" {
            # "Why did I do a GUID here?"
            # "Template Separator\n(You can make a copy of, or modify, this frame)"
            n165 = Unbundle By Name(w425) -> ("PopSubpanel"=w433:i32, "Self Reference"=w431:refnum<class "SMO.UI.MAUI.lvclass">)
            n166 = Unbundle By Name(w431) -> ("Subpanels"=w434:refnum<class "SMO.UI.Embedded.lvclass">[])
            n167 = Index Array(array=w434, index=w433) -> (element=w432:refnum<class "SMO.UI.Embedded.lvclass">)
            n168 = call <vilib>:"GetGUID.vi"("error in (no error)"=w427, "SMO"=w432) -> ("error out"=w429:errorcluster, "GUID"=w430:string)  [unwired: 7 in, 1 out]
            n169 = call "OpenSubpanelHandler.vi"("error in (no error)"=w429, "GUID"=w430, "SMO.UI.MAUI in"=w431) -> ("error out"=w428:errorcluster, "SMO.UI.MAUI out"=w424:refnum<class "SMO.UI.MAUI.lvclass">)  [unwired: 7 in]
            n170 = Bundle By Name(cluster=w425, "Self Reference"=w424) -> (w426:T9)
            n171 = call <vilib>:"Add State(s) to Queue__jki_lib_state_machine.vi"("State(s) in (\"\")"=w437) -> ("States Out"=w436:string)  [unwired: 14 in]
          }
          frame "Framework: UI State" {
            # "Template Separator\n(You can make a copy of, or modify, this frame)"
            n172 = Unbundle By Name(w439) -> ("Self Reference"=w445:refnum<class "SMO.UI.MAUI.lvclass">, "UI State"=w443:T8)
            n173 = call "HandleStateChange.vi"("error in (no error)"=w441, "UI State"=w443, "GUID"=w444, "SMO.UI.MAUI in"=w445) -> ("error out"=w442:errorcluster, "SMO.UI.MAUI out"=w438:refnum<class "SMO.UI.MAUI.lvclass">)  [unwired: 6 in]
            n174 = Bundle By Name(cluster=w439, "Self Reference"=w438) -> (w440:T9)
            n175 = call <vilib>:"Add State(s) to Queue__jki_lib_state_machine.vi"("State(s) in (\"\")"=w448) -> ("States Out"=w447:string)  [unwired: 14 in]
          }
          frame "Framework: Update Panel" {
            # "Changes Embedded in Subpanel\n(Based on panel index and active index values)"
            n176 = Unbundle By Name(w455) -> ("Self Reference"=w456:refnum<class "SMO.UI.MAUI.lvclass">, "Panel Index"=w450:i32[], "Active Index"=w449:i32[])
            n177 = for {
              tunnel: w456 -> [w465]
              tunnel: [w464] -> w453
              shift-right: [w462] -> w451
              shift-left: w452 -> [w463]
              tunnel: w450 -> [w461] mode=indexing
              tunnel: w449 -> [w460] mode=indexing
              n178 = call "ChangePanel.vi"("error in (no error)"=w463, "New Active Index"=w460, "Panel Index"=w461, "MAUI in"=w465) -> ("error out"=w462:errorcluster, "MAUI out"=w464:refnum<class "SMO.UI.MAUI.lvclass">)  [unwired: 6 in]
            }
            n179 = Bundle By Name(cluster=w455, "Self Reference"=w453) -> (w454:T9)
            n180 = call <vilib>:"Add State(s) to Queue__jki_lib_state_machine.vi"("State(s) in (\"\")"=w459) -> ("States Out"=w458:string)  [unwired: 14 in]
          }
          frame "Framework: Grey Rings" {
            # "Greys all taken values except the one in current ring\n(Call this after panel has been updated)"
            n181 = Unbundle By Name(w467) -> ("Self Reference"=w471:refnum<class "SMO.UI.MAUI.lvclass">)
            n182 = call "GreyRings.vi"("error in (no error)"=w470, "MAUI in"=w471) -> ("error out"=w469:errorcluster, "MAUI out"=w468:refnum<class "SMO.UI.MAUI.lvclass">)  [unwired: 8 in]
            n183 = Bundle By Name(cluster=w467, "Self Reference"=w468) -> (w466:T9)
            n184 = call <vilib>:"Add State(s) to Queue__jki_lib_state_machine.vi"("State(s) in (\"\")"=w474) -> ("States Out"=w473:string)  [unwired: 14 in]
          }
          frame "Framework: Populate Rings" {
            # "Writes string array to ring controls"
            n185 = Unbundle By Name(w479) -> ("Self Reference"=w480:refnum<class "SMO.UI.MAUI.lvclass">)
            n186 = call "PopulateRings.vi"("error in (no error)"=w476, "MAUI in"=w480) -> ("error out"=w475:errorcluster, "MAUI out"=w477:refnum<class "SMO.UI.MAUI.lvclass">)  [unwired: 8 in]
            n187 = Bundle By Name(cluster=w479, "Self Reference"=w477) -> (w478:T9)
            n188 = call <vilib>:"Add State(s) to Queue__jki_lib_state_machine.vi"("State(s) in (\"\")"=w483) -> ("States Out"=w482:string)  [unwired: 14 in]
          }
        }
      }
    }
    frame Error {
    }
  }
  n189 = call-parent "Process.vi"("error in (no error)"=w8, "SMO.UI"=w7) -> ("error out"=w5:errorcluster, "SMO.UI out"=→"MAUI out":refnum<class "SMO.UI.MAUI.lvclass">)  [unwired: 8 in]
  n190 = Merge Errors(w5, w4) -> (→"error out":errorcluster)
